vi "读取我的属性和方法.vi"(8 "error in (no error)":errorcluster caption="错误输入（无错误）", 11 "鸭子输入":refnum<class "鸭子.lvclass">) -> (0 "error out":errorcluster caption="错误输出", 2 "我的属性和方法":string, 3 "鸭子输出":refnum<class "鸭子.lvclass">)   [LabVIEW 2022 SP3, in "鸭子库.lvlib" / "鸭子.lvclass"]
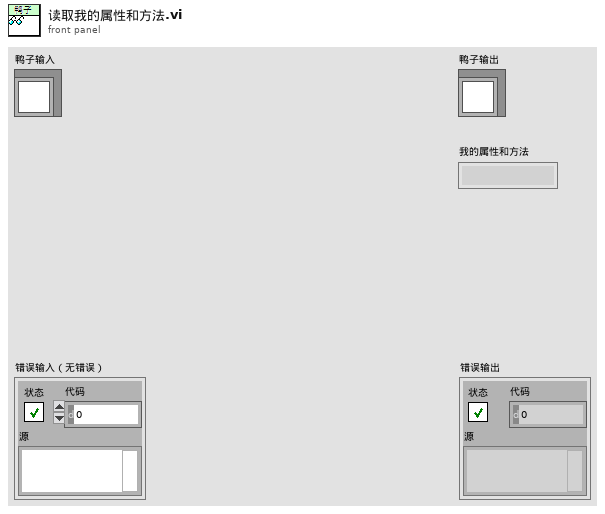
[diagram p1: front panel]
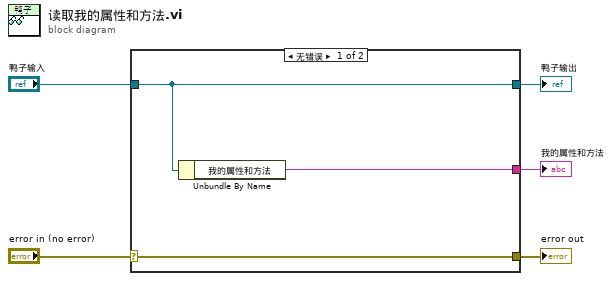
[diagram p0: block diagram]
diagram:
  n1 = case shown="无错误" "error in (no error)" {
    selector: "error in (no error)" -> [w8 w9]
    tunnel: [w8 w9] -> w4
    tunnel: [w7 w10] -> w2
    tunnel: "鸭子输入" -> [w7 w10]
    tunnel: [w6 _] -> w1
    frame No Error {
      n2 = Unbundle By Name(w7) -> ("我的属性和方法"=w6:string)
    }
    frame Error {
    }
  }
  "error out" <- w4
  "鸭子输出" <- w2
  "我的属性和方法" <- w1
